vi "Process.vi"(11 "Actor":refnum<class "Error Handler Actor.lvclass">) -> ()   [LabVIEW 2021, in "Error Handler Actor.lvclass"]
uses:
  Error Handler Actor.lvclass
  Error Handler Actor.lvclass/Error Handler Actor.ctl
  Re-use Libraries/Utility/Utility.lvlib
  Re-use Libraries/Minimal Actor Framework/Actors/Base Actor/Actor/Front Panel State.ctl
  Re-use Libraries/Minimal Actor Framework/Actors/Base Actor/Actor/Actor.lvclass
  Re-use Libraries/Minimal Actor Framework/Messaging/Message/Message.lvclass
  Re-use Libraries/Utility/UI/System Button (without mouse hover).ctl
panel:
  out "Errors":errorcluster[](array[cluster])
  in  "Acknowledge":T1
  out "Number Of Errors":i32
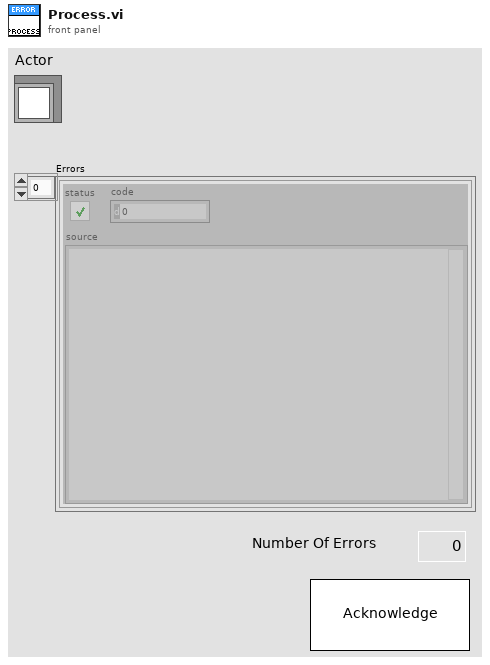
[diagram p1: front panel]
types:
  T1 = typedef "Utility.lvlib/System Button (without mouse hover).ctl" = bool
  T2 = typedef "Actor.lvclass/Front Panel State.ctl" = enum32{"Invalid", "Standard", "Closed", "Hidden", "Minimized", "Maximized"}
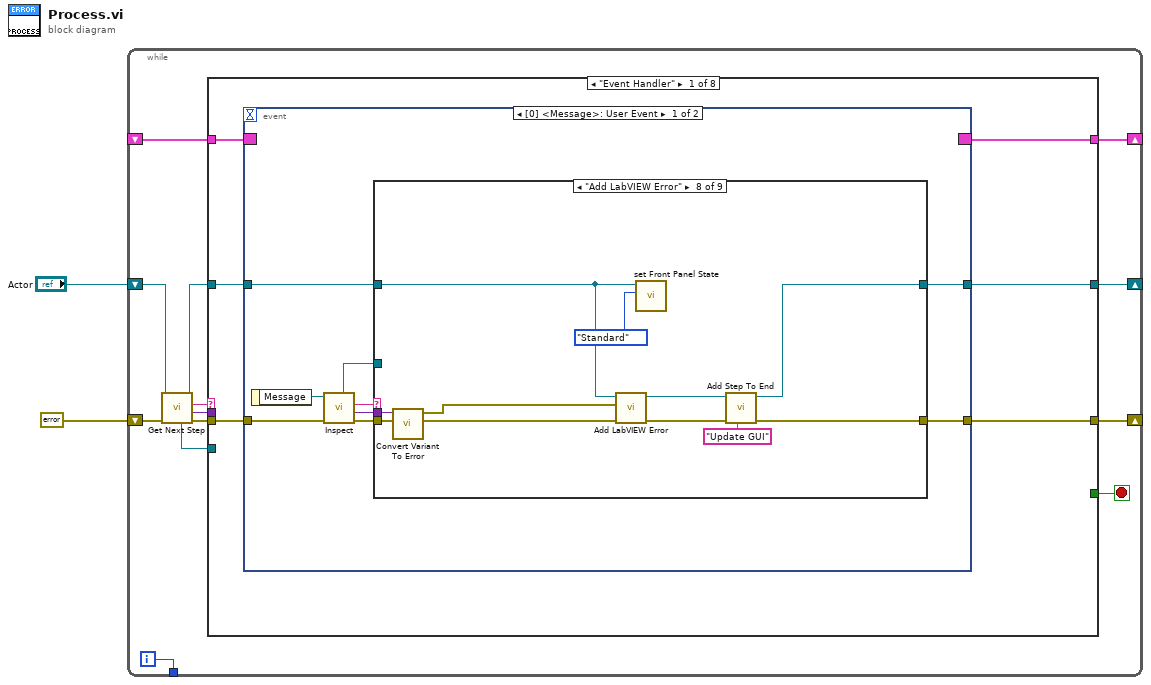
[diagram p0: block diagram]
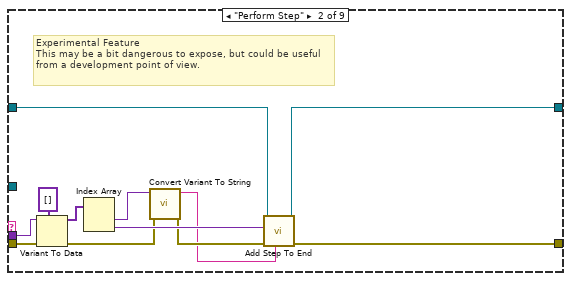
[diagram p3: hidden frame]
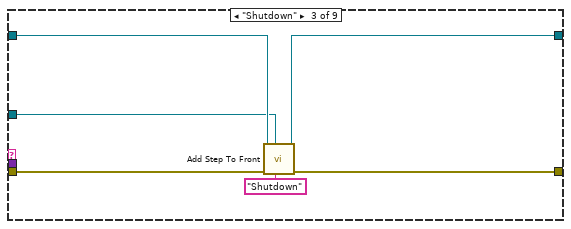
[diagram p4: hidden frame]
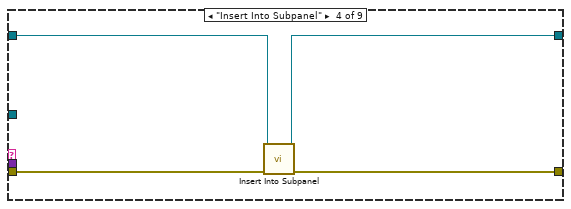
[diagram p5: hidden frame]
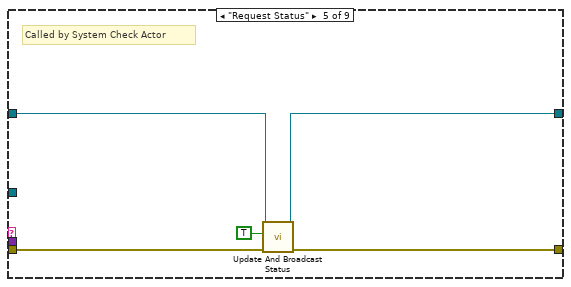
[diagram p6: hidden frame]
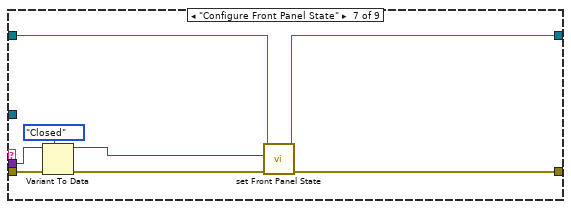
[diagram p8: hidden frame]
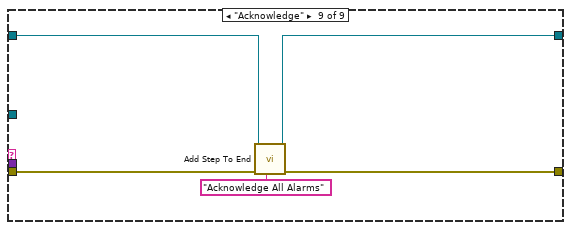
[diagram p9: hidden frame]
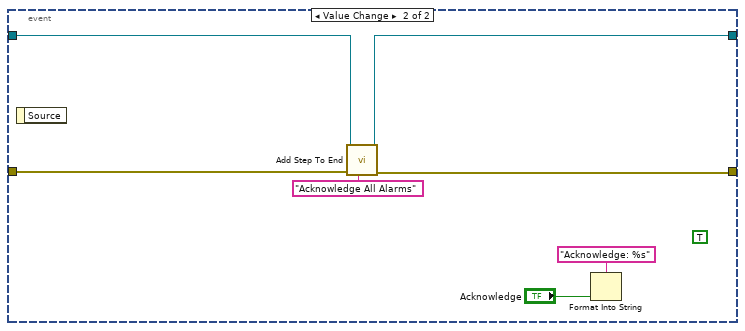
[diagram p10: hidden frame]
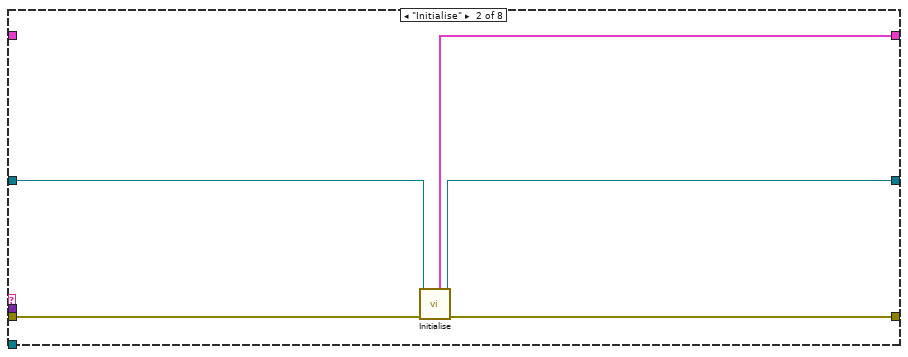
[diagram p11: hidden frame]
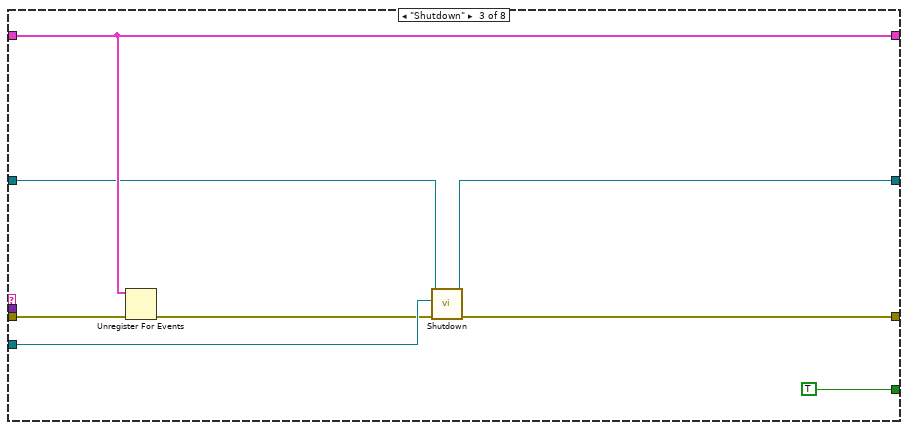
[diagram p12: hidden frame]
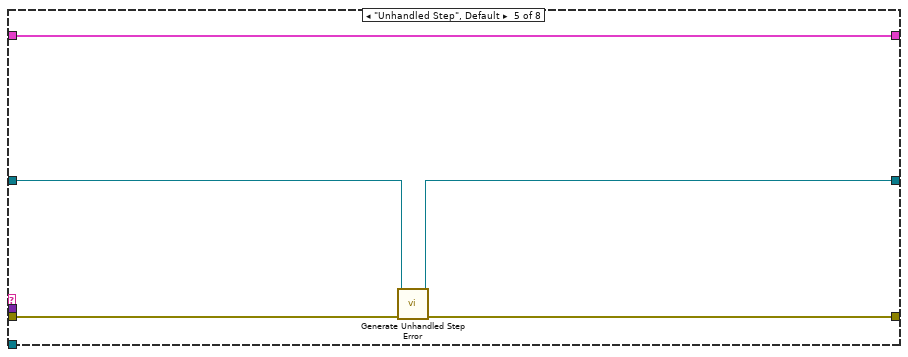
[diagram p14: hidden frame]
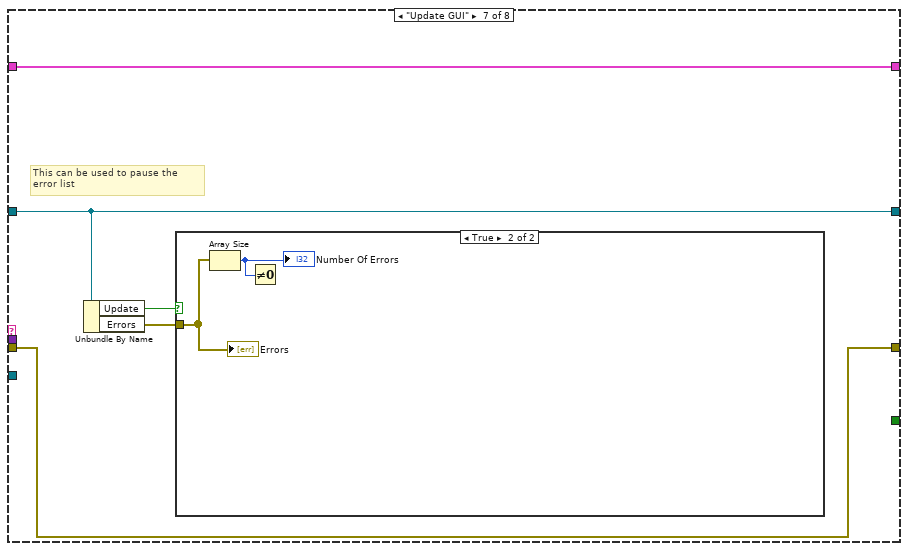
[diagram p16: hidden frame]
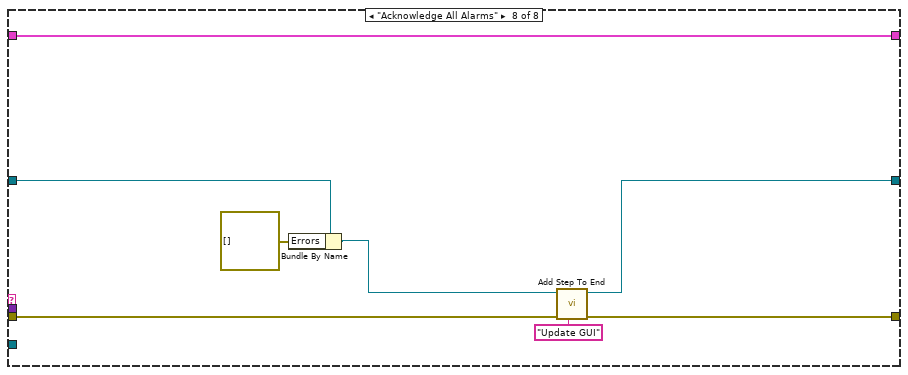
[diagram p18: hidden frame]
diagram:
  n1 = while {
    shift-right: [w4] -> _
    shift-left: "Actor" -> [w3]
    shift-right: [w11] -> _
    shift-left: _ -> [w10]
    shift-right: [w8] -> _
    shift-left: errorcluster {"status"=FALSE, "code"=0, "source"=""} ("error constant") -> [w7]
    tunnel: [w6] -> _
    i -> [w6]
    stop <- w15 stop-if-true
    n2 = call-dynamic "Get Next Step.vi"("error in (no error)"=w7, "Actor in"=w3) -> ("error out"=w9:errorcluster, "Parameter"=w12:variant, "Step"=w13:string, "Actor out"=w14:refnum<class "Error Handler Actor.lvclass">, "Reply Channel"=w5:refnum<notifier>)  [unwired: 5 in]
    n3 = case shown="\"Event Handler\"" w13 {
      tunnel: [_ _ TRUE _ _ _ _ _] -> w15
      tunnel: w14 -> [w21 w97 w99 w106 w112 w114 w118 w127]
      tunnel: [w16 w93 w101 w106 w109 w114 w118 w128] -> w4
      tunnel: w12 -> [_ _ _ _ _ _ _ _]
      tunnel: [w19 w94 w104 w108 w113 w116 w121 w131] -> w11
      tunnel: w10 -> [w20 _ w104 w108 w113 w116 w121 w131]
      tunnel: w9 -> [w18 w96 w103 w107 w111 w115 w117 w125]
      tunnel: [w17 w95 w102 w107 w110 w115 w117 w129] -> w8
      tunnel: w5 -> [_ _ w100 _ _ _ _ _]
      frame "Event Handler" {
        n4 = event shown="[0] <Message>: User Event" {
          selector: w20 -> [_ _]
          dyn-events: [_ _] -> w19
          timeout: _ -> [_ _]
          tunnel: w21 -> [w30 w89]
          tunnel: [w29 w86] -> w16
          tunnel: w18 -> [w27 w92]
          tunnel: [w28 w88] -> w17
          event User Event {
            n5 = event-data() -> ("Message"=w26:refnum<class "Message.lvclass">)  [unwired: 1 in]
            n6 = call "Inspect.vi"("error in (no error)"=w27, "Message in"=w26) -> ("error out"=w23:errorcluster, "Data"=w24:variant, "Name"=w25:string, "Reply Channel"=w22:refnum<notifier>)  [unwired: 5 in, 1 out]
            n7 = case shown="\"Add LabVIEW Error\"" w25 {
              tunnel: w30 -> [w32 w44 w50 w54 w58 w60 w69 w71 w85]
              tunnel: [w32 w43 w49 w53 w57 w60 w68 w72 w81] -> w29
              tunnel: w23 -> [w31 w41 w47 w52 w56 w61 w65 w80 w84]
              tunnel: [w31 w42 w46 w51 w55 w61 w67 w74 w82] -> w28
              tunnel: w24 -> [_ w33 _ _ _ _ w66 w79 _]
              tunnel: w22 -> [_ _ w45 _ _ _ _ _ _]
              frame Default {
              }
              frame "Perform Step" {
                # "Experimental Feature\nThis may be a bit dangerous to expose, but could be useful from a development point of view."
                n8 = Variant To Data(error in=w41, type=variant[] [], Variant=w33) -> (data=w39:variant[], error out=w36:errorcluster)
                n9 = Index Array(array=w39) -> (element #1=w37:variant, element #2=w38:variant)  [unwired: 2 in]
                n10 = call "Convert Variant To String.vi"("error in (no error)"=w36, "Variant"=w37) -> ("error out"=w35:errorcluster, "String"=w34:string)  [unwired: 8 in]
                n11 = call-dynamic "Add Step To End.vi"("Step Name"=w34, "error in (no error)"=w35, "Parameter"=w38, "Actor in"=w44) -> ("error out"=w42:errorcluster, "Actor out"=w43:refnum<class "Error Handler Actor.lvclass">)  [unwired: 6 in]
              }
              frame "Shutdown" {
                n12 = call-dynamic "Add Step To Front.vi"("Step Name"="Shutdown", "Reply Channel"=w45, "error in (no error)"=w47, "Actor in"=w50) -> ("error out"=w46:errorcluster, "Actor out"=w49:refnum<class "Error Handler Actor.lvclass">)  [unwired: 6 in]
              }
              frame "Insert Into Subpanel" {
                n13 = call-dynamic "Insert Into Subpanel.vi"("error in (no error)"=w52, "Actor in"=w54) -> ("error out"=w51:errorcluster, "Actor out"=w53:refnum<class "Error Handler Actor.lvclass">)  [unwired: 8 in]
              }
              frame "Request Status" {
                # "Called by System Check Actor"
                n14 = call-dynamic "Update And Broadcast Status.vi"("error in (no error)"=w56, "OK"=TRUE, "Actor in"=w58) -> ("error out"=w55:errorcluster, "Actor out"=w57:refnum<class "Error Handler Actor.lvclass">)  [unwired: 7 in]
              }
              frame "State Update Tick" {
                # "Metronome is not used in Alarm Handler.\n\nNo action here. Look at the System Check actor"
                # "Called by the Metronome"
              }
              frame "Configure Front Panel State" {
                n15 = Variant To Data(error in=w65, type=Front_Panel_State."Closed" ("Front Panel State"), Variant=w66) -> (data=w62:T2, error out=w64:errorcluster)
                n16 = call-dynamic "set Front Panel State.vi"("error in (no error)"=w64, "Front Panel State"=w62, "Actor in"=w69) -> ("error out"=w67:errorcluster, "Actor out"=w68:refnum<class "Error Handler Actor.lvclass">)  [unwired: 7 in]
              }
              frame "Add LabVIEW Error" {
                n17 = call "Convert Variant To Error.vi"("error in (no error)"=w80, "Variant"=w79) -> ("error out"=w77:errorcluster, "Error"=w78:errorcluster)  [unwired: 8 in]
                n18 = call "Add LabVIEW Error.vi"("error in (no error)"=w77, "LabVIEW Error"=w78, "Alarm Handler Actor in"=w71) -> ("error out"=w75:errorcluster, "Alarm Handler Actor out"=w73:refnum<class "Error Handler Actor.lvclass">)  [unwired: 7 in]
                n19 = call-dynamic "set Front Panel State.vi"("Front Panel State"=Front_Panel_State."Standard", "Actor in"=w71) -> ()  [unwired: 8 in, 2 out]
                n20 = call-dynamic "Add Step To End.vi"("Step Name"="Update GUI", "error in (no error)"=w75, "Actor in"=w73) -> ("error out"=w74:errorcluster, "Actor out"=w72:refnum<class "Error Handler Actor.lvclass">)  [unwired: 7 in]
              }
              frame "Acknowledge" {
                n21 = call-dynamic "Add Step To End.vi"("Step Name"="Acknowledge All Alarms", "error in (no error)"=w84, "Actor in"=w85) -> ("error out"=w82:errorcluster, "Actor out"=w81:refnum<class "Error Handler Actor.lvclass">)  [unwired: 7 in]
              }
            }
          }
          event Value Change {
            (unwired) TRUE
            n22 = event-data() -> ()  [unwired: 1 in, 1 out]
            n23 = call-dynamic "Add Step To End.vi"("Step Name"="Acknowledge All Alarms", "error in (no error)"=w92, "Actor in"=w89) -> ("error out"=w88:errorcluster, "Actor out"=w86:refnum<class "Error Handler Actor.lvclass">)  [unwired: 7 in]
            n24 = Format Into String(format string="Acknowledge: %s", "Acknowledge") -> ()  [unwired: 2 in, 2 out]
          }
        }
      }
      frame "Initialise" {
        n25 = call "Initialise.vi"("error in (no error)"=w96, "Actor in"=w97) -> ("error out"=w95:errorcluster, "Actor out"=w93:refnum<class "Error Handler Actor.lvclass">, "Observers"=w94:cluster{"Actor":refnum<event-registration>})  [unwired: 7 in]
      }
      frame "Shutdown" {
        n26 = Unregister For Events(event registration refnum=w104, error in=w103) -> (error out=w98:errorcluster)
        n27 = call-dynamic "Shutdown.vi"("error in (no error)"=w98, "Reply Channel"=w100, "Actor in"=w99) -> ("error out"=w102:errorcluster, "Actor out"=w101:refnum<class "Error Handler Actor.lvclass">)  [unwired: 7 in]
      }
      frame "Error Handler" {
        # "Don't really want the error handler to add more errors!\n\nHopefully this state will never occur."
      }
      frame "Unhandled Step", Default {
        n28 = call-dynamic "Generate Unhandled Step Error.vi"("error in (no error)"=w111, "Actor in"=w112) -> ("error out"=w110:errorcluster, "Actor out"=w109:refnum<class "Error Handler Actor.lvclass">)  [unwired: 8 in]
      }
      frame "-----------------------" {
        # "Separator"
      }
      frame "Update GUI" {
        # "This can be used to pause the error list"
        n29 = Unbundle By Name(w118) -> ("Update"=w119:bool, "Errors"=w120:errorcluster[])
        n30 = case shown="True" w119 {
          tunnel: w120 -> [_ w123]
          frame False {
          }
          frame True {
            n31 = Array Size(array=w123) -> (size(s)=w122:i32)
            "Number Of Errors" <- w122
            n32 = Not Equal To 0?(x=w122) -> ()  [unwired: 1 out]
            "Errors" <- w123
          }
        }
      }
      frame "Acknowledge All Alarms" {
        n33 = Bundle By Name(cluster=w127, "Errors"=errorcluster[] []) -> (w126:refnum<class "Error Handler Actor.lvclass">)
        n34 = call-dynamic "Add Step To End.vi"("Step Name"="Update GUI", "error in (no error)"=w125, "Actor in"=w126) -> ("error out"=w129:errorcluster, "Actor out"=w128:refnum<class "Error Handler Actor.lvclass">)  [unwired: 7 in]
      }
    }
  }
